vi "SSOFC测试系统.vi"() -> ()   [LabVIEW 2019]
doc: "This example shows how to configure the instrument's output voltage level, over current protection, and over voltage protection. The actual voltage level and actual current level are returned as well as whether over voltage protection (OVP) or over current protection (OCP) has been tripped."
uses:
  <vilib>/Utility/file.llb/Write Delimited Spreadsheet (DBL).vi
  <instrlib>/PSW/PSW.lvlib
panel:
  out "(NL/h)":dbl
  out "产氢速率 (NL/h)":dbl(graph)
  in  "电解模式 开/关":bool
  out "I (A)":dbl
  out "U (V)":dbl
  out "P(W)":dbl
  out "输出功率 P (W)":dbl(graph)
  out "电流 I (A)":dbl(graph)
  in  "数据保存路径":path=path "D:/labview/Output.xls"
  out "电压 U (V)":dbl(graph)
  out "CC":bool
  out "?":bool
  in  "保护电流 (A)":dbl=36.0 format="%.3g"
  in  "Serial Configuration":T1={"Baud Rate"=9600, "Parity"=0, "Data Bits"=8, "Stop Bits"=10, "Flow Control"=0} {"Flow Control" items=["None", "XON/XOFF", "RTS/CTS", "XON/XOFF & RTS/CTS", "DTR/DSR", "XON/XOFF & DTR/DSR"]; "Stop Bits" items=["1.0"=10, "1.5"=15, "2.0"=20]; "Data Bits" items=["7"=7, "8"=8]; "Parity" items=["None", "Odd", "Even", "Mark", "Space"]; "Baud Rate" items=["300"=300, "600"=600, "1200"=1200, "2400"=2400, "4800"=4800, "9600"=9600, "19200"=19200]}
  in  "Stop Output":bool
  out "OCP Tripped?":bool
  out "OVP Tripped?":bool
  in  "保护电压 (V)":dbl=30.0 format="%.3f"
  out "电流 (A)":dbl format="%.3f"
  out "电压 (V)":dbl format="%.3f"
  in  "电势 E (V)":dbl=21.0 format="%.3f"
  in  "电流上限 (A)":dbl=35.0 format="%.3f"
  in  "通道":refnum<visa-resource-name>="COM3"
  # "可逆固体氧化物电池综合能源系统测试平台"
  # "电压 U"
  # "电流 I"
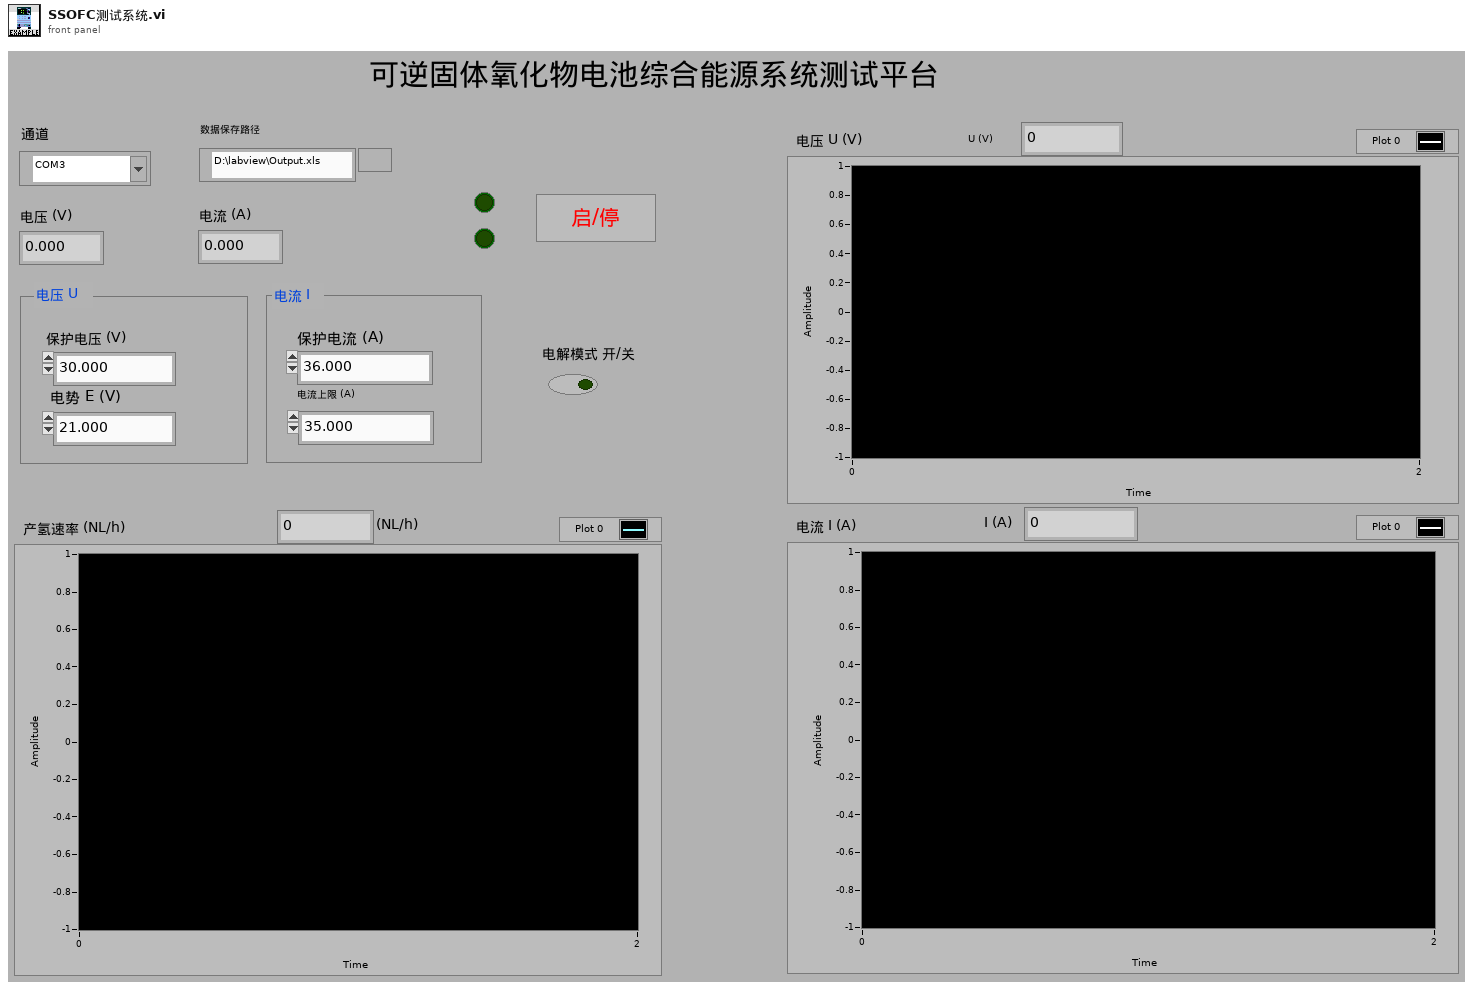
[diagram p1: front panel]
types:
  T1 = cluster{"Baud Rate":u32, "Parity":u16, "Data Bits":u16, "Stop Bits":u16, "Flow Control":u16}
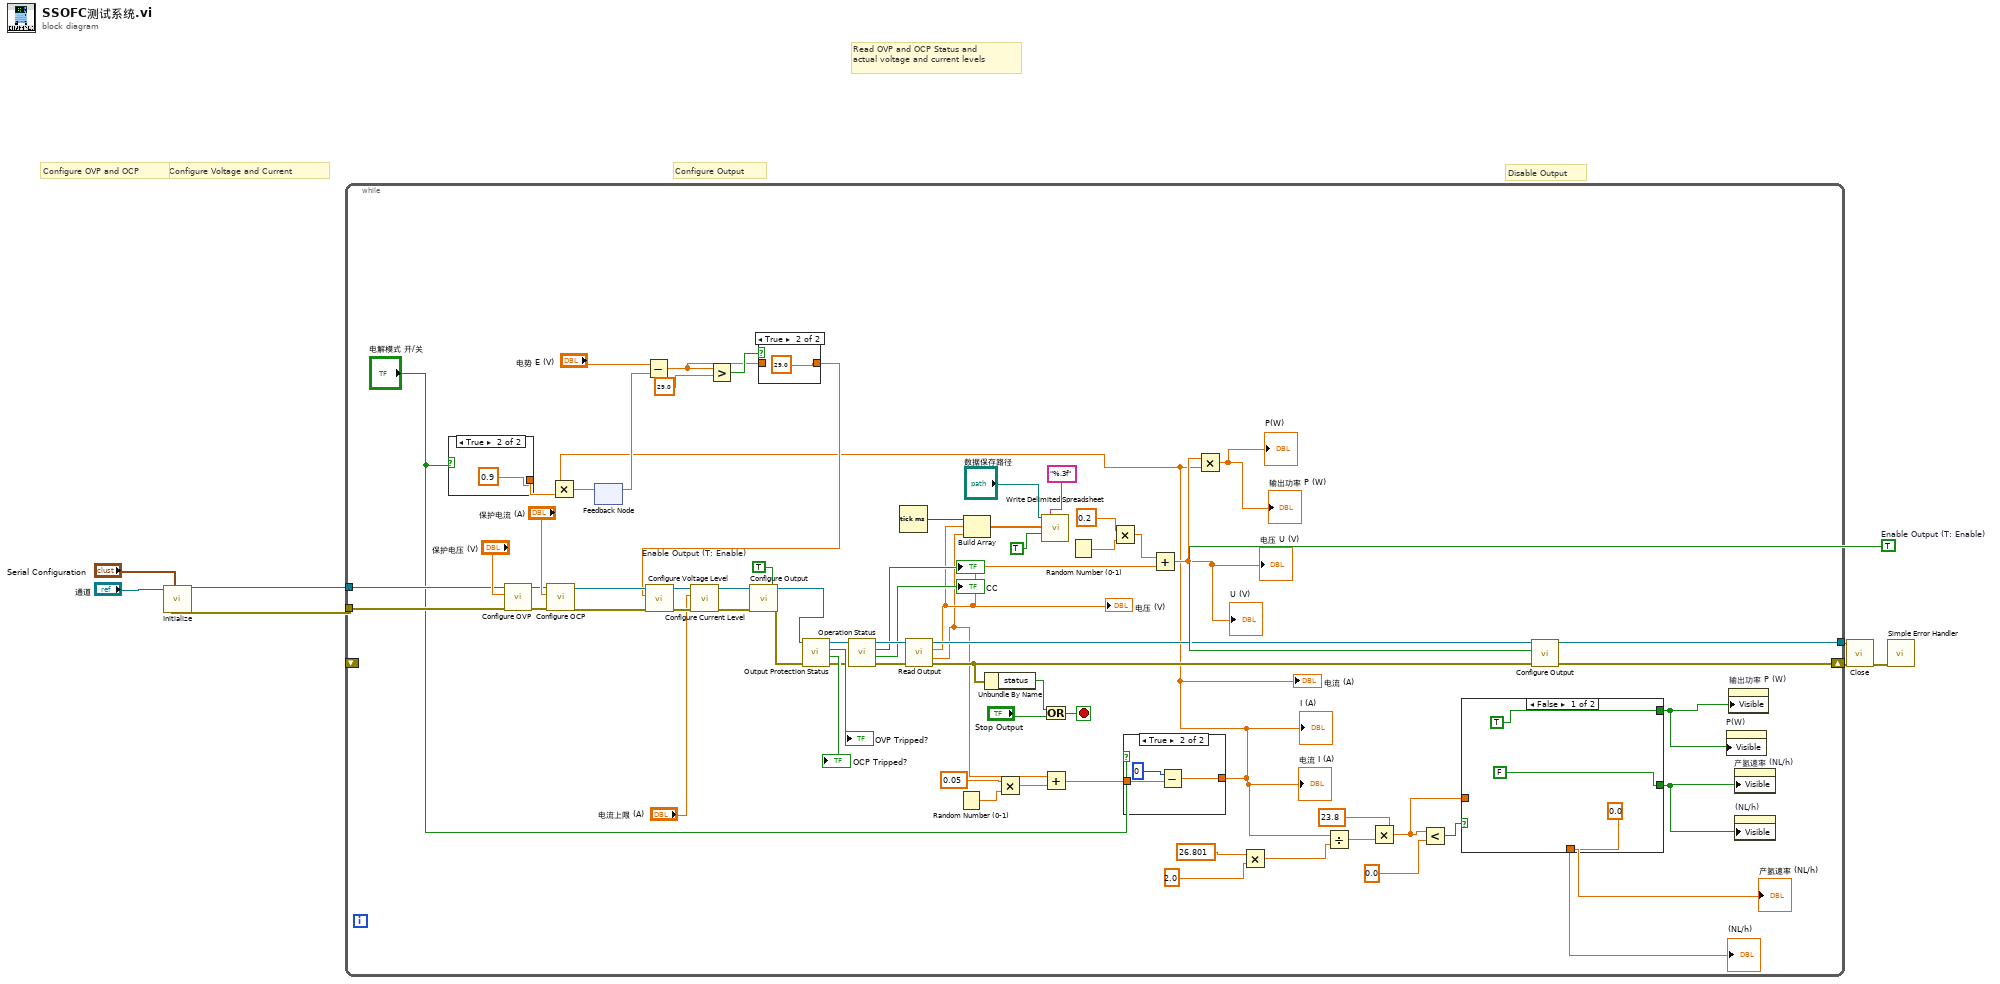
[diagram p0: block diagram]
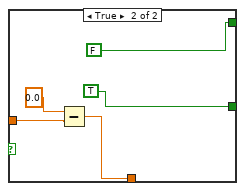
[diagram p2: hidden frame]
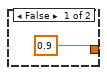
[diagram p5: hidden frame]
diagram:
  w3 = TRUE  # Enable Output (T: Enable)
  # "Configure Voltage and Current"
  # "Disable Output"
  # "Read OVP and OCP Status and\nactual voltage and current levels"
  # "Configure Output"
  # "Configure OVP and OCP"
  n1 = call <instrlib>:"Initialize.vi"("Serial Configuration"="Serial Configuration", "VISA resource name"="通道") -> ("error out"=w2:errorcluster, "VISA resource name out"=w1:refnum<visa-resource-name>)  [unwired: 3 in, 5 out]
  n2 = while {
    tunnel: [w76] -> w9
    shift-right: [w71] -> w8
    shift-left: _ -> [_]
    tunnel: w2 -> [w50]
    tunnel: w1 -> [w49]
    stop <- w73 stop-if-true
    w51 = TRUE  # Enable Output (T: Enable)
    n3 = case shown="True" "电解模式 开/关" {
      tunnel: [0.9 0.9] -> w32
      frame False {
      }
      frame True {
      }
    }
    n4 = call <instrlib>:"Configure OVP.vi"("error in (no error)"=w50, "OVP (0.000 V)"="保护电压 (V)", "VISA resource name"=w49) -> ("error out"=w53:errorcluster, "VISA resource name out"=w54:refnum<visa-resource-name>)  [unwired: 2 in, 5 out]
    n5 = call <instrlib>:"Configure OCP.vi"("error in (no error)"=w53, "OCP (0.000 V)"="保护电流 (A)", "VISA resource name"=w54) -> ("error out"=w57:errorcluster, "VISA resource name out"=w56:refnum<visa-resource-name>)  [unwired: 7 out]
    n6 = feedback #1() -> (w27:dbl)  [unwired: 1 in]
    n7 = Subtract(x="电势 E (V)", y=w27) -> (x-y=w23:dbl)
    n8 = Greater?(x=w23, y=29.0) -> (0:w26:bool)
    n9 = case shown="True" w26 {
      tunnel: [w85 29.0] -> w24
      tunnel: w23 -> [w85 _]
      frame False {
      }
      frame True {
      }
    }
    n10 = call <instrlib>:"Configure Voltage Level.vi"("error in (no error)"=w57, "Voltage Level (0.000 V)"=w24, "VISA resource name"=w56) -> ("error out"=w59:errorcluster, "VISA resource name out"=w58:refnum<visa-resource-name>)  [unwired: 7 out]
    n11 = call <instrlib>:"Configure Current Level.vi"("error in (no error)"=w59, "Current Level (0.000 A)"="电流上限 (A)", "VISA resource name"=w58) -> ("error out"=w61:errorcluster, "VISA resource name out"=w60:refnum<visa-resource-name>)  [unwired: 7 out]
    n12 = call <instrlib>:"Configure Output.vi"("error in (no error)"=w61, "Enable Output (T: Enable)"=w51, "VISA resource name"=w60) -> ("error out"=w47:errorcluster, "VISA resource name out"=w48:refnum<visa-resource-name>)  [unwired: 2 in, 5 out]
    n13 = call <instrlib>:"Output Protection Status.vi"("error in (no error)"=w47, "VISA resource name"=w48) -> ("error out"=w68:errorcluster, "OCP Tripped?"=→"OCP Tripped?":bool, "OVP Tripped?"=→"OVP Tripped?":bool, "VISA resource name out"=w69:refnum<visa-resource-name>)  [unwired: 1 in, 5 out]
    n14 = call <instrlib>:"Operation Status.vi"("error in (no error)"=w68, "VISA resource name"=w69) -> ("error out"=w66:errorcluster, "CC"=→"CC":bool, "CV"=→"?":bool, "VISA resource name out"=w67:refnum<visa-resource-name>)  [unwired: 6 out]
    n15 = Tick Count (ms)() -> (millisecond timer value=w45:u32)
    n16 = call <instrlib>:"Read Output.vi"("error in (no error)"=w66, "VISA resource name"=w67) -> ("error out"=w71:errorcluster, "Actual Current Level (A)"=w35:dbl, "Actual Voltage Level (V)"=w43:dbl, "VISA resource name out"=w76:refnum<visa-resource-name>)  [unwired: 1 in, 5 out]
    "电压 (V)" <- w43
    n17 = Random Number (0-1)() -> (number: 0 to 1=w37:dbl)
    n18 = Build Array(w45, w43, w35) -> (w62:dbl[])
    n19 = Unbundle By Name(w71) -> ("status"=w70:bool)
    n20 = Multiply(x=0.05, y=w37) -> (x*y=w36:dbl)
    n21 = call-poly <vilib>:"Write Delimited Spreadsheet.vi"("file path (dialog if empty)"="数据保存路径", "format (%.3f)"="%.3f", "1D data"=w62, "append to file? (new file:F)"=TRUE) -> ()  [unwired: 10 in, 2 out]
    n22 = Or(x=w70, y="Stop Output") -> (x .or. y?=w73:bool)
    n23 = Add(x=w35, y=w36) -> (x+y=w29:dbl)
    n24 = Random Number (0-1)() -> (number: 0 to 1=w41:dbl)
    n25 = Multiply(x=0.2, y=w41) -> (x*y=w39:dbl)
    n26 = case shown="True" "电解模式 开/关" {
      tunnel: w29 -> [w87 w89]
      tunnel: [w87 w88] -> w20
      frame False {
      }
      frame True {
        n27 = Subtract(x=0, y=w89) -> (x-y=w88:dbl)
      }
    }
    "电流 (A)" <- w20
    "电流 I (A)" <- w20
    "I (A)" <- w20
    n28 = Multiply(x=w20, y=w32) -> (x*y=w31:dbl)
    n29 = feedback-in #1(w31) -> ()
    n30 = Add(x=w39, y=w43) -> (x+y=w33:dbl)
    "电压 U (V)" <- w33
    "U (V)" <- w33
    n31 = Multiply(x=w33, y=w20) -> (x*y=→"输出功率 P (W)" →"P(W)":dbl)
    n32 = Multiply(x=26.801, y=2.0) -> (x*y=w19:dbl)
    n33 = Divide(x=w20, y=w19) -> (x/y=w18:dbl)
    n34 = Multiply(x=23.8, y=w18) -> (x*y=w14:dbl)
    n35 = Less?(x=w14, y=0.0) -> (x < y?=w16:bool)
    n36 = case shown="False" w16 {
      tunnel: [0.0 w82] -> w13
      tunnel: w14 -> [_ w83]
      tunnel: [FALSE TRUE] -> w12
      tunnel: [TRUE FALSE] -> w11
      frame False {
      }
      frame True {
        n37 = Subtract(x=0.0, y=w83) -> (x-y=w82:dbl)
      }
    }
    "产氢速率 (NL/h)" <- w13
    "(NL/h)" <- w13
    n38 = property on="P(W)" class="DigNum (strict)"("Visible"=w11) -> ()  [unwired: 2 in, 2 out]
    n39 = property on="输出功率 P (W)" class="WFChart (strict)"("Visible"=w11) -> ()  [unwired: 2 in, 2 out]
    n40 = property on="产氢速率 (NL/h)" class="WFChart (strict)"("Visible"=w12) -> ()  [unwired: 2 in, 2 out]
    n41 = property on="(NL/h)" class="DigNum (strict)"("Visible"=w12) -> ()  [unwired: 2 in, 2 out]
  }
  n42 = call <instrlib>:"Configure Output.vi"("error in (no error)"=w8, "Enable Output (T: Enable)"=w3, "VISA resource name"=w9) -> ("error out"=w6:errorcluster, "VISA resource name out"=w7:refnum<visa-resource-name>)  [unwired: 1 in, 6 out]
  n43 = call <instrlib>:"Close.vi"("error in (no error)"=w6, "VISA resource name"=w7) -> ("error out"=w5:errorcluster)  [unwired: 9 out]
  n44 = call <vilib>:"Simple Error Handler.vi"("error in (no error)"=w5) -> ()  [unwired: 1 in, 8 out]
